vi "getMode.vi"(8 "error in (no error)":errorcluster, 11 "Inst.FP in":refnum<class "Inst.FP.lvclass">) -> (0 "error out":errorcluster, 2 "Mode":T1, 3 "Inst.FP out":refnum<class "Inst.FP.lvclass">)   [LabVIEW 2019, in "Inst.FP.lvclass"]
doc: "Gets the current operating <b>Mode</b> of the GHS."
uses:
  Inst.FP.lvclass
  C:/Program Files (x86)/National Instruments/LabVIEW 2019/user.lib/LevyLab/Instrument Framework/SMOs/Instrument/Instrument.lvclass
  Typedefs/Inst.FP.Modes--Enum.ctl
  Typedefs/Inst.FP.Get Mode--Cluster.ctl
  Typedefs/Inst.FP.Commands--Enum.ctl
  <userlib>/LevyLab/Instrument Framework/SMOs/Instrument/Instrument.lvclass/Instrument.ctl
  d5aeea22-43ef-4aeb-99ea-2317f764c5f3.vi
  d5aeea22-43ef-4aeb-99ea-2317f764c5f3.vi/03e54a4b-02c8-4ac7-8f31-c79cfd90bcdf.vi
  <userlib>/LevyLab/Instrument Framework/SMOs/Instrument/API/Send and Receive.vi
  d5aeea22-43ef-4aeb-99ea-2317f764c5f3.vi/f7a10209-7759-4223-8391-e2e1b1c6c3f5.vi
  <userlib>/LevyLab/Instrument Framework/SMOs/Instrument/Private/Get Client Type.vi
  d5aeea22-43ef-4aeb-99ea-2317f764c5f3.vi/03e54a4b-02c8-4ac7-8f31-c79cfd90bcdf.vi/42db3566-277f-480c-bcf1-8cab9a3181c9.vi
  d5aeea22-43ef-4aeb-99ea-2317f764c5f3.vi/03e54a4b-02c8-4ac7-8f31-c79cfd90bcdf.vi/ade40c86-aec6-4fd7-aa2c-940876ceea9f.vi
  d5aeea22-43ef-4aeb-99ea-2317f764c5f3.vi/f7a10209-7759-4223-8391-e2e1b1c6c3f5.vi/4e71f28f-30d7-4fb3-a20a-1481ac80578b.vi
  d5aeea22-43ef-4aeb-99ea-2317f764c5f3.vi/f7a10209-7759-4223-8391-e2e1b1c6c3f5.vi/d671af2b-e81a-46a5-8e78-80af1c55d245.vi
  d5aeea22-43ef-4aeb-99ea-2317f764c5f3.vi/f7a10209-7759-4223-8391-e2e1b1c6c3f5.vi/4e71f28f-30d7-4fb3-a20a-1481ac80578b.vi/aa65acd6-10e7-4c89-ba94-feee2dd0eeb2.vi
  d5aeea22-43ef-4aeb-99ea-2317f764c5f3.vi/f7a10209-7759-4223-8391-e2e1b1c6c3f5.vi/4e71f28f-30d7-4fb3-a20a-1481ac80578b.vi/49430cc3-b0fe-41fd-ae62-d5b2a85f9db4.vi
  <userlib>/LevyLab/Instrument Framework/SMOs/Instrument/Private/Get RC Connection Status.vi
  <userlib>/LevyLab/Instrument Framework/SMOs/Instrument/API/Enum to String.vi
  <userlib>/LevyLab/Instrument Framework/SMOs/RemoteControl/API/Send and Receive.vi
  <vilib>/Utility/Data Type/Get Type Information.vi
  <vilib>/JDP Science/JSONtext/JSON text to Variant.vi
  <userlib>/LevyLab/Instrument Framework/SMOs/Instrument/API/Instrument.GetPublicEvents.vi
  <vilib>/JDP Science/JSONtext/Variant to JSON Text.vi
  <vilib>/National Instruments/GUID Generator/Guid Generator.vi
  <userlib>/LevyLab/Instrument Framework/SMOs/Instrument/API/Instrument.MessageToProcess.vi
  <userlib>/LevyLab/Instrument Framework/SMOs/Instrument/Private/Instrument.MessageFromProcess.EventStructure.vi
  <vilib>/JDP Science/JSONtext/LVClass Serializer/JSONtext LVClass Serializer.lvclass
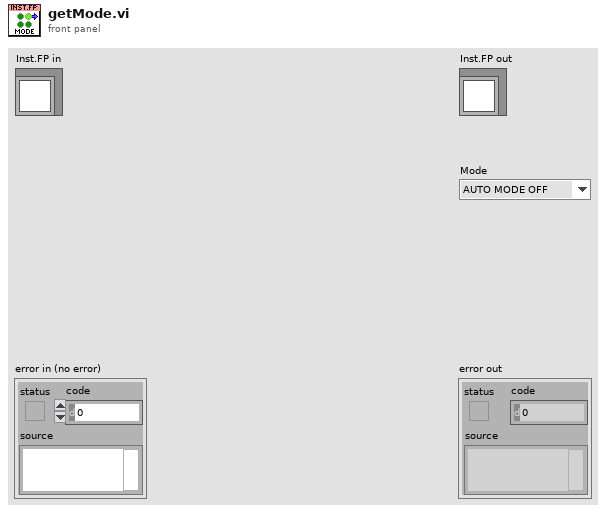
[diagram p1: front panel]
types:
  T1 = typedef "Inst.FP.lvclass/Inst.FP.Modes--Enum.ctl" = enum16{"AUTO MODE OFF", "START", "CONDENSING 3He", "CONDENSING 4He", "NORMAL CIRCULATION", "RECOVERY OF THE MIXTURE", "RECOVERY: BLOCKAGE or OVERPRESSURE"}
  T2 = typedef "Inst.FP.lvclass/Inst.FP.Commands--Enum.ctl" = enum16{"getMode", "setMode", "pushButton"}
  T3 = typedef "Inst.FP.lvclass/Inst.FP.Get Mode--Cluster.ctl" = cluster{"Mode":T1}
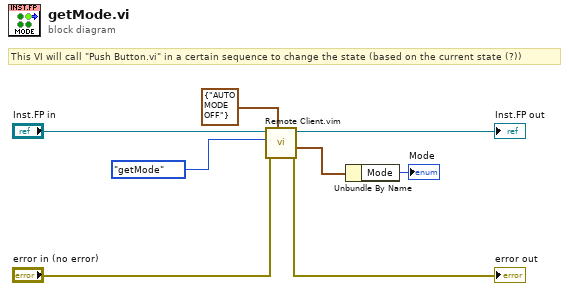
[diagram p0: block diagram]
diagram:
  # "This VI will call \"Push Button.vi\" in a certain sequence to change the state (based on the current state (?))"
  n1 = call "Remote Client.vim"("Data Out type"=T3 {"Mode"=enum."AUTO MODE OFF"} ("Get Mode"), "error in (no error)"="error in (no error)", "method"=Inst.FP.Commands--Enum."getMode" ("Commands"), "Instrument in"="Inst.FP in") -> ("error out"=→"error out":errorcluster, "Data out"=w2:T3, "Instrument out"=→"Inst.FP out":refnum<class "Inst.FP.lvclass">)  [unwired: 4 in, 1 out]
  n2 = Unbundle By Name(w2) -> ("Mode"=→"Mode":T1)
